vi "Robot Main.vi"() -> ()   [LabVIEW 2012]
doc: "This VI imlements the framework and scheduler for your robotics program. It should not be necessary to modify the framework. You are expected to add your code to the VIs called from Robot Main, the ones located in the Team Code within the project."
uses:
  <vilib>/Rock Robotics/WPI/Camera/WPI_CameraImageSize.ctl
  Robot Global Data.vi
panel:
  out "Timings":cluster{"Call Name":string, "Delta (ms)":u32}[](array[cluster])
  in  "Image Size":T1=enum."160x120"
  in  "Finish":bool
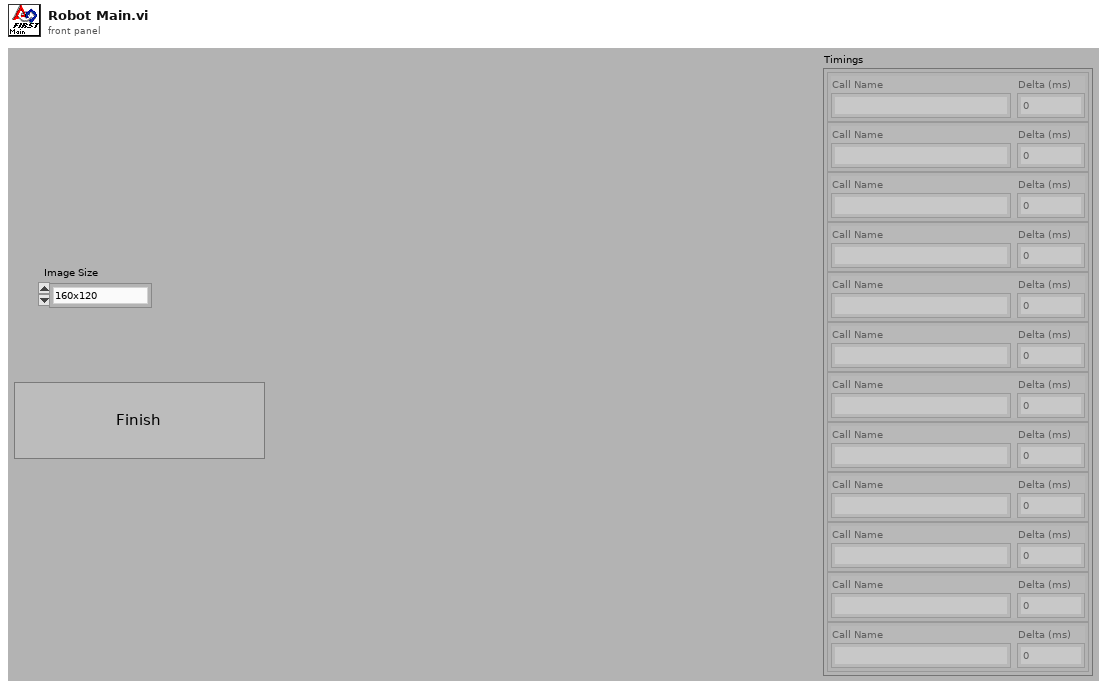
[diagram p1: front panel]
types:
  T1 = typedef "WPI_CameraImageSize.ctl" = enum16{"640x480", "320x240", "160x120"}
  T2 = typedef "WPI_DriverStationMatch Info.ctl" = cluster{"Autonomous Elapsed Seconds":dbl, "TeleOp Elapsed Seconds":dbl, "Disabled Elapsed Seconds":dbl, "Visited Autonomous":bool, "Visited TeleOp":bool, "Visited Disabled":bool, "Autonomous Settings":cluster{"Autonomous Style":enum16{"Iterative", "Independent"}, "VI Refnum":refnum<vi>}}
  T3 = typedef "WPI_DriverStationDerivedRobotMode.ctl" = enum16{"Init", "Execute", "Stop"}
  T4 = typedef "WPI_DriverStationRobotMode2.ctl" = enum16{"Autonomous Disabled", "Autonomous Enabled", "Teleop Disabled", "Teleop Enabled", "Timeout", "Finish", "Test Disabled", "Test Enabled"}
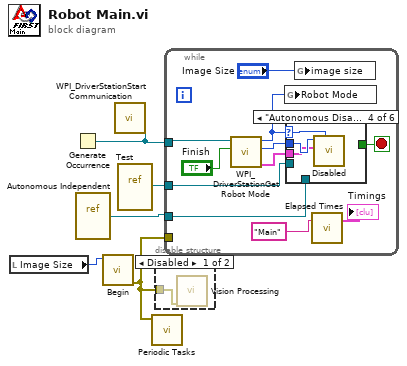
[diagram p0: block diagram]
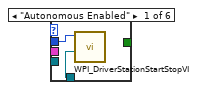
[diagram p3: hidden frame]
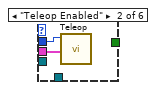
[diagram p4: hidden frame]
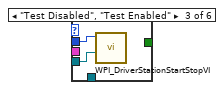
[diagram p5: hidden frame]
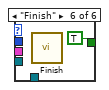
[diagram p7: hidden frame]
diagram:
  n1 = local read "Image Size"() -> (w2:T1)
  n2 = Generate Occurrence() -> (w5:refnum<k4>)
  n3 = vi-ref "Autonomous Independent.vi"() -> (w4:refnum<vi>)
  n4 = call "Begin.vi"("Image Size"=w2) -> ("error out"=w1:errorcluster)  [unwired: 10 out]
  n5 = call <vilib>:"WPI_DriverStationStart Communication.vi"("occurrence"=w5) -> ()  [unwired: 11 out]
  n6 = vi-ref "Test.vi"() -> (w3:refnum<vi>)
  n7 = call "Periodic Tasks.vi"("error in (no error)"=w1) -> ()  [unwired: 1 in, 10 out]
  n8 = disable-structure shown="Disabled" {
    disable-tunnel: w1 -> [w6 _]
    frame Disabled {
      n9 = call "Vision Processing.vi"("error in (no error)"=w6) -> ()  [unwired: 3 in, 4 out]
    }
    frame Enabled {
    }
  }
  n10 = while "Scheduling loop" {
    tunnel: w5 -> [w16]
    tunnel: w4 -> [w12]
    tunnel: w3 -> [w10]
    tunnel: w1 -> [_]
    stop <- w13 stop-if-true
    n11 = call <vilib>:"WPI_DriverStationGet Robot Mode.vi"("Finish"="Finish", "DS Occurrence"=w16) -> ("Match Info out"=w14:T2, "Call Context"=w17:T3, "Robot Mode"=w9:T4)  [unwired: 7 out]
    n12 = global write "Robot Global Data.vi" "Robot Mode"(w9) -> ()
    n13 = case shown="\"Autonomous Disabled\", \"Teleop Disabled\"" w9 {
      selector: w9 -> [_ _ _ w24 _ _]
      tunnel: w17 -> [w19 w21 w23 w26 _ _]
      tunnel: w14 -> [_ w20 _ w25 _ _]
      tunnel: [_ _ _ _ _ TRUE] -> w13
      tunnel: w12 -> [w18 _ _ _ _ _]
      tunnel: w10 -> [_ _ w22 _ _ _]
      frame "Autonomous Enabled" {
        n14 = call <vilib>:"WPI_DriverStationStartStopVI.vi"("VI in"=w18, "Call Context"=w19) -> ()  [unwired: 10 in]
      }
      frame "Teleop Enabled" {
        n15 = call "Teleop.vi"("Match Info"=w20, "Call Context"=w21) -> ()  [unwired: 1 in, 9 out]
      }
      frame "Test Disabled", "Test Enabled" {
        n16 = call <vilib>:"WPI_DriverStationStartStopVI.vi"("VI in"=w22, "Call Context"=w23) -> ()  [unwired: 10 in]
      }
      frame "Autonomous Disabled", "Teleop Disabled" {
        n17 = call "Disabled.vi"("Robot Mode"=w24, "Match Info"=w25, "Call Context"=w26) -> ()  [unwired: 1 in, 8 out]
      }
      frame "Timeout" {
      }
      frame "Finish" {
        n18 = call "Finish.vi"() -> ()  [unwired: 1 in, 7 out]
      }
    }
    n19 = global write "Robot Global Data.vi" "image size"("Image Size") -> ()
    n20 = call "Elapsed Times.vi"("Call Name"="Main") -> ("Timings"=→"Timings":cluster{"Call Name":string, "Delta (ms)":u32}[])  [unwired: 2 in]
  }
